vi "find_point_in_tables.vi"(8 "T No.":enum16{"0", "1", "2", "3", "4"}(ring), 9 "T Search":dbl, 10 "P Search":dbl) -> (3 "Point":T7)   [LabVIEW 2017]
uses:
  <vilib>/Utility/file.llb/Read Delimited Spreadsheet (DBL).vi
panel:
  out "all rows":dbl[][](array[numeric])
  out "appended path":path
  out "P Search 2":dbl
  out "T Founded":dbl
  out "Super_Heated_T_Curves":T1(ring)
  out "Super_Heated_S_Curves":enum16{"P", "S", "H gas"}(ring)
  out "Super_Heated_T_Curves 2":T2
  out "Super_Heated_S_Curves 2":T3
  out "Sat_Deg_10_Step":T4(ring)
  out "Sat_Deg_10_Step 2":T5
  out "Sat_By_Deg":T4(ring)
  out "Sat_By_Deg 2":T6
  out "Saturation Degrees( 10 Steps )":dbl[][](array[numeric])
  out "Super_Heated_S_Curves 3":dbl[][](array[numeric])
  out "Super_Heated_T":dbl[][](array[numeric])
  out "T Search Index In Sat Table":dbl
  out "Sat_By_Deg_Arr":dbl[][](array[numeric])
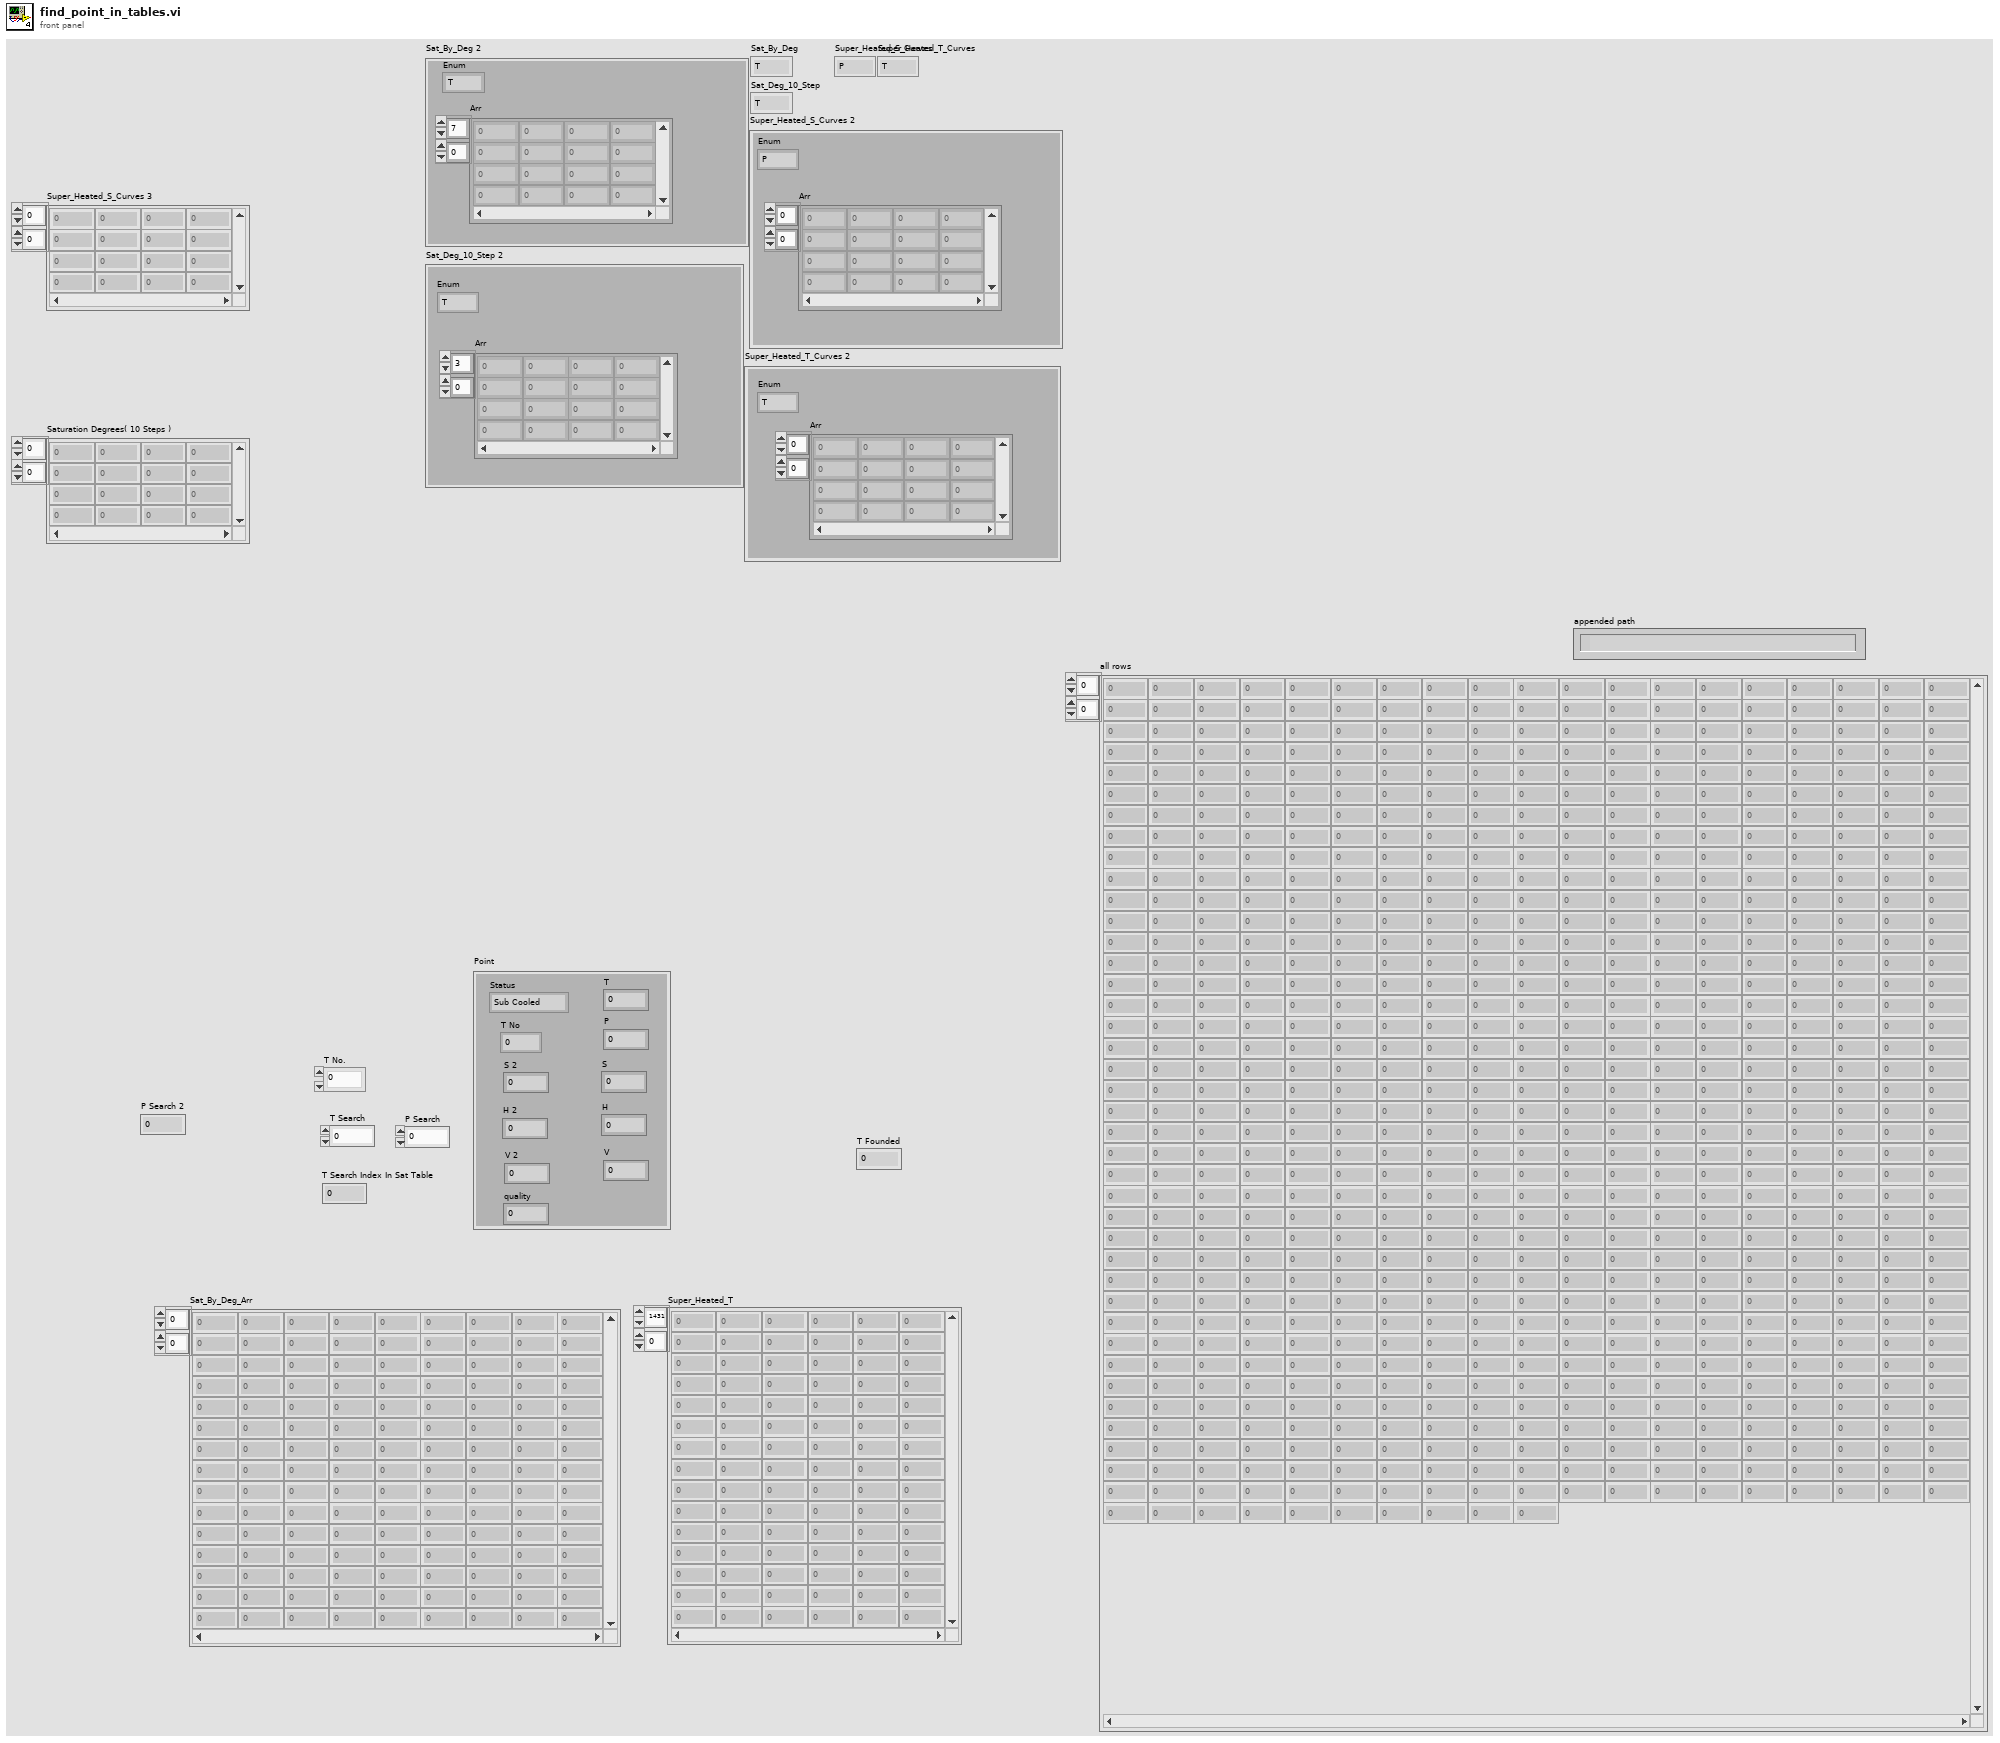
[diagram p1: front panel]
types:
  T1 = enum16{"T", "P", "T_Sat_Vapor", "Hg", "Sg", "Vg"}
  T2 = cluster{"Enum":enum16{"T", "P", "T_Sat_Vapor", "Hg", "Sg", "Vg"}, "Arr":dbl[][]}
  T3 = cluster{"Enum":enum16{"P", "S", "H gas"}, "Arr":dbl[][]}
  T4 = enum16{"T", "P", "V1", "Vg", "H1", "Hg", "R", "S1", "Sg"}
  T5 = cluster{"Enum":enum16{"T", "P", "V1", "Vg", "H1", "Hg", "R", "S1", "Sg"}, "Arr":dbl[][]}
  T6 = cluster{"Enum":enum16{"T", "P", "V1", "Vg", "H1", "Hg", "R", "S1", "Sg"}, "Arr ":dbl[][]}
  T7 = cluster{"S":dbl, "H":dbl, "V":dbl, "T":dbl, "P":dbl, "Status":enum16{"Sub Cooled", "Saturation", "Super Heated"}, "S 2":dbl, "H 2":dbl, "V 2":dbl, "T No":enum16{"0", "1", "2", "3", "4"}, "quality":dbl}
  T8 = enum16{"Sub Cooled", "Saturation", "Super Heated"}
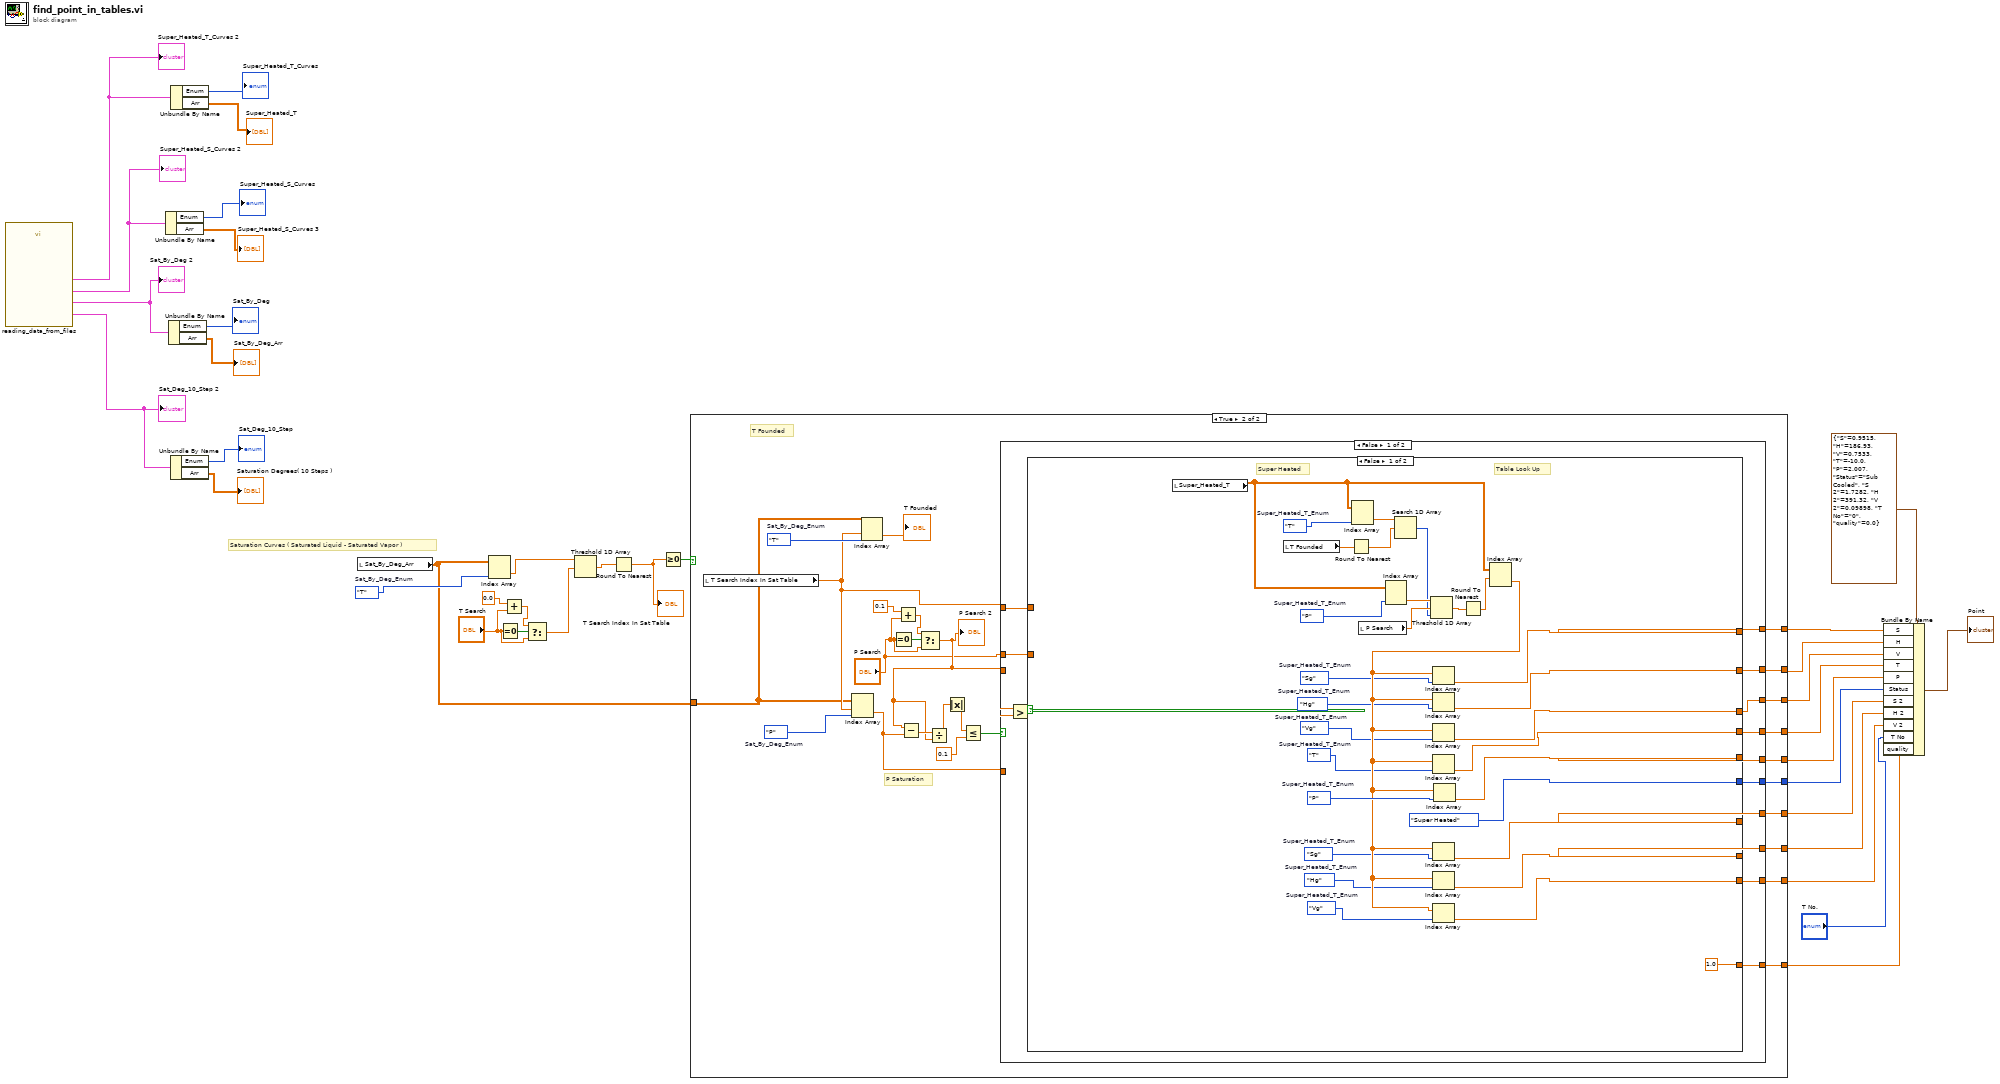
[diagram p0: block diagram]
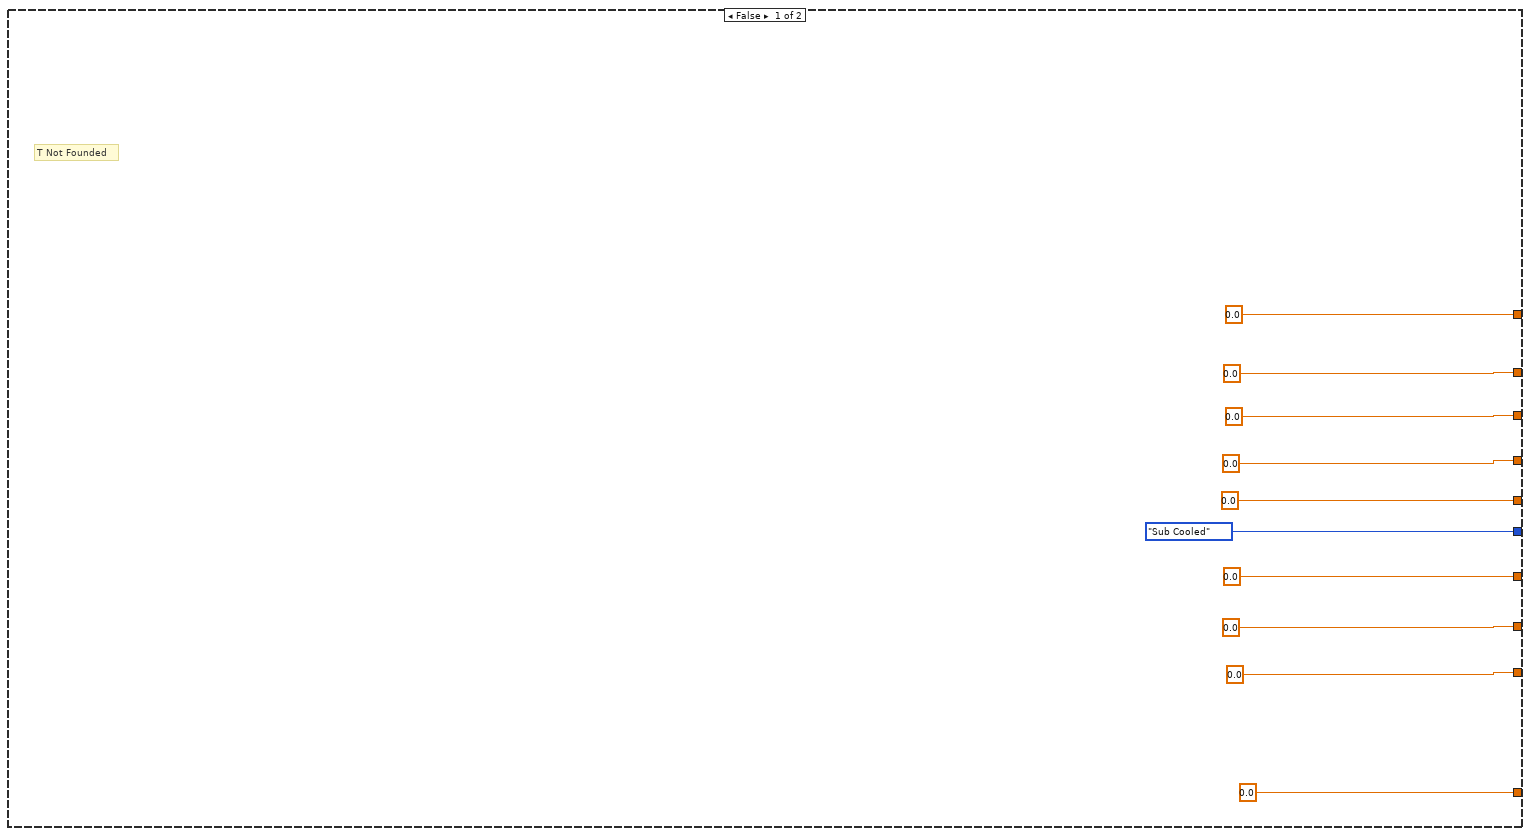
[diagram p2: hidden frame]
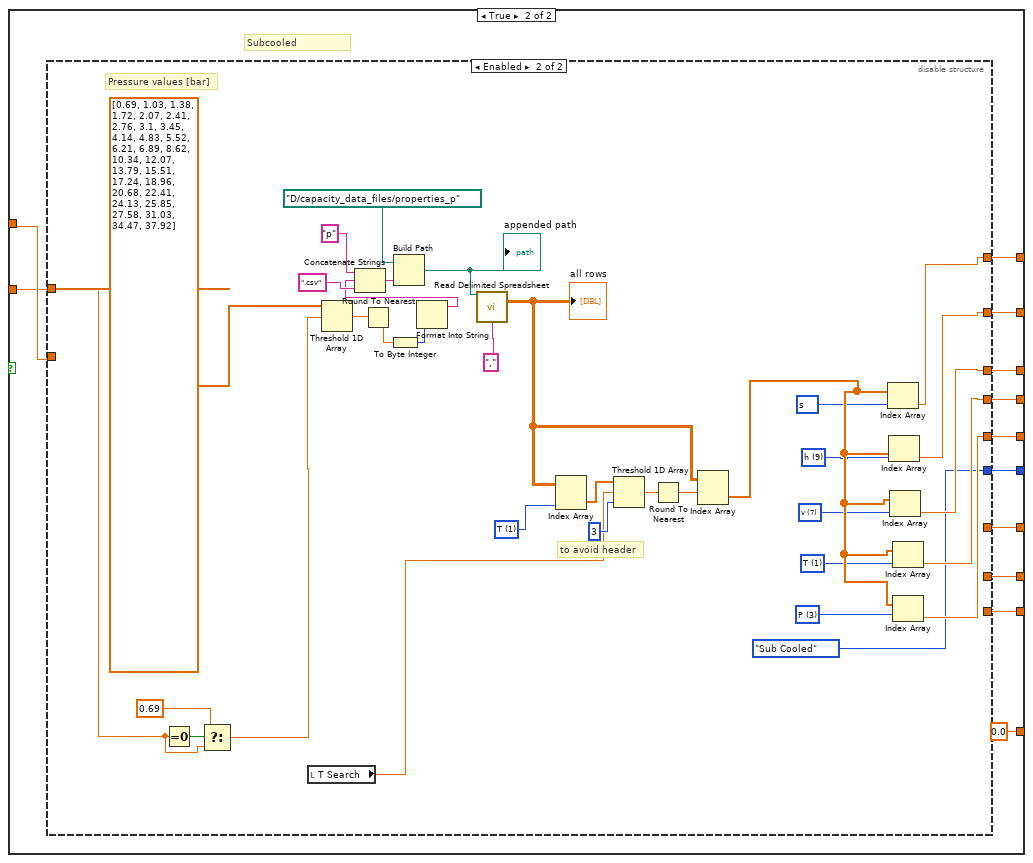
[diagram p3: hidden frame]
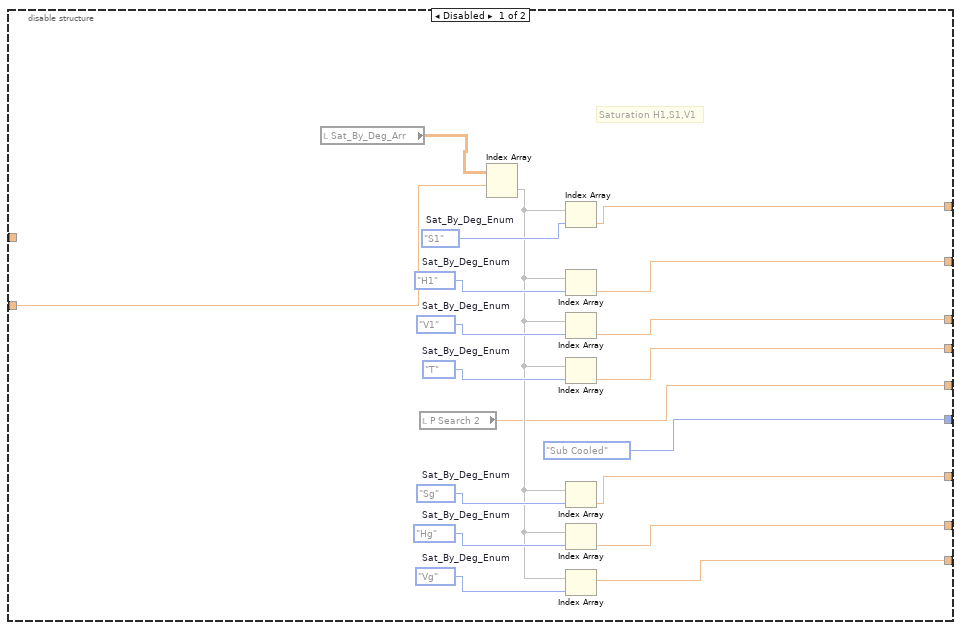
[diagram p4: hidden frame]
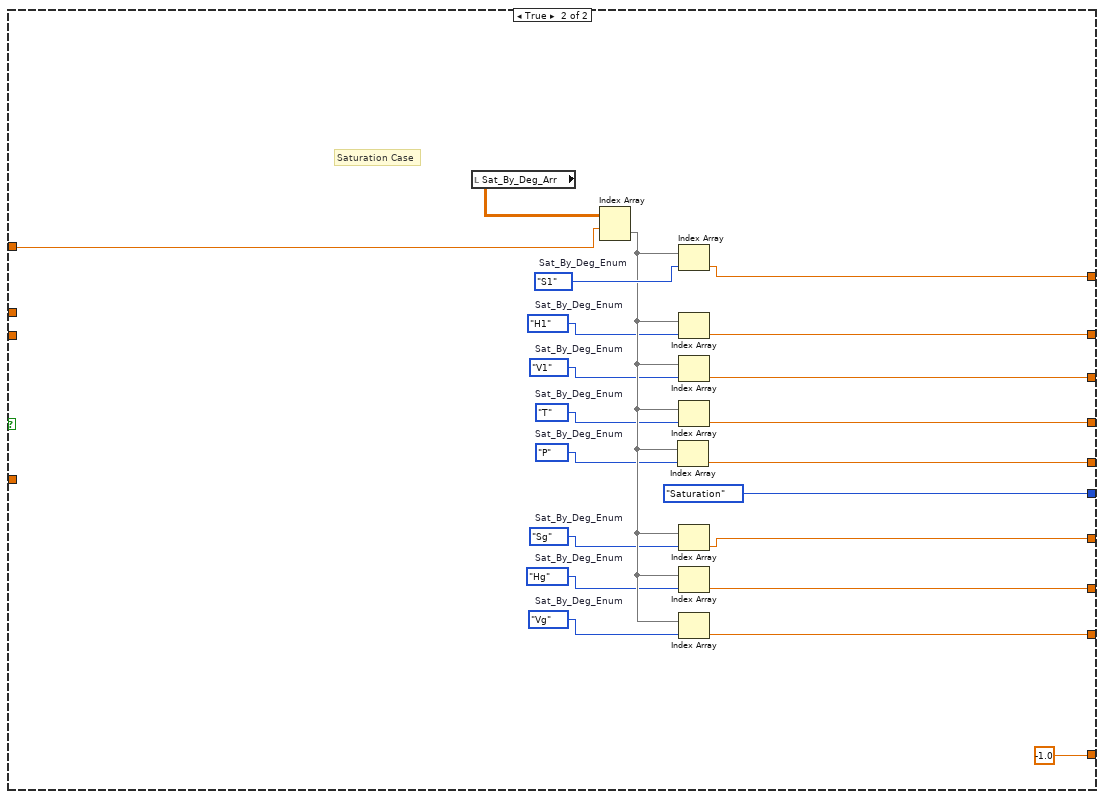
[diagram p5: hidden frame]
diagram:
  w34 = T4."T"  # Sat_By_Deg_Enum
  # "Saturation Curves ( Saturated Liquid - Saturated Vapor )"
  n1 = call "reading_data_from_files.vi"() -> ("Super_Heated_T_Curves"=w14:T2, "Super_Heated_S_Curves"=w15:T3, "Sat_Deg_10_Step"=w18:T5, "Sat_By_Deg"=w20:T6)  [unwired: 8 in]
  "Sat_By_Deg 2" <- w20
  "Sat_Deg_10_Step 2" <- w18
  "Super_Heated_S_Curves 2" <- w15
  "Super_Heated_T_Curves 2" <- w14
  n2 = Unbundle By Name(w15) -> ("Enum"=→"Super_Heated_S_Curves":enum16{"P", "S", "H gas"}, "Arr"=→"Super_Heated_S_Curves 3":dbl[][])
  n3 = Unbundle By Name(w20) -> ("Enum"=→"Sat_By_Deg":T4, "Arr"=→"Sat_By_Deg_Arr":dbl[][])
  n4 = Unbundle By Name(w18) -> ("Enum"=→"Sat_Deg_10_Step":T4, "Arr"=→"Saturation Degrees( 10 Steps )":dbl[][])
  n5 = Unbundle By Name(w14) -> ("Enum"=→"Super_Heated_T_Curves":T1, "Arr"=→"Super_Heated_T":dbl[][])
  n6 = local read "Sat_By_Deg_Arr"() -> (w22:dbl[][])
  n7 = Index Array(array=w22, index (col)=w34) -> (element=w24:dbl[])  [unwired: 1 in]
  n8 = Equal To 0?(x="T Search") -> (x = 0?=w7:bool)
  n9 = Add(x=0.0, y="T Search") -> (x+y=w6:dbl)
  n10 = Select(t=w6, s=w7, f="T Search") -> (s? t:f=w3:dbl)
  n11 = Threshold 1D Array(2:w3, 3:w24) -> (0:w23:dbl)  [unwired: 1 in]
  n12 = Round To Nearest(number=w23) -> (nearest integer value=w21:dbl)
  "T Search Index In Sat Table" <- w21
  n13 = Greater Or Equal To 0?(x=w21) -> (x >= 0?=w36:bool)
  n14 = case shown="True" w36 {
    tunnel: [0.0 ("Numeric") w72] -> w33
    tunnel: [0.0 ("Numeric") w71] -> w32
    tunnel: [0.0 ("Numeric") w70] -> w31
    tunnel: [0.0 ("Numeric") w69] -> w30
    tunnel: [0.0 ("Numeric") w68] -> w29
    tunnel: [0.0 ("Numeric") w67] -> w28
    tunnel: [0.0 ("Numeric") w66] -> w27
    tunnel: [0.0 ("Numeric") w65] -> w26
    tunnel: [T8."Sub Cooled" ("Status") w64] -> w25
    tunnel: w22 -> [_ w57]
    tunnel: [0.0 w47] -> w1
    frame False {
      # "T Not Founded"
    }
    frame True {
      w59 = T4."T"  # Sat_By_Deg_Enum
      w63 = T4."P"  # Sat_By_Deg_Enum
      # "P Saturation"
      # "T Founded"
      n15 = local read "T Search Index In Sat Table"() -> (w58:dbl)
      n16 = Index Array(array=w57, index (row)=w58, index (col)=w63) -> (element=w60:dbl)
      n17 = Index Array(array=w57, index (row)=w58, index (col)=w59) -> (element=→"T Founded":dbl)
      n18 = Equal To 0?(x="P Search") -> (x = 0?=w52:bool)
      n19 = Add(x=0.1, y="P Search") -> (x+y=w51:dbl)
      n20 = Select(t=w51, s=w52, f="P Search") -> (s? t:f=w49:dbl)
      "P Search 2" <- w49
      n21 = Subtract(x=w49, y=w60) -> (x-y=w55:dbl)
      n22 = Divide(x=w55, y=w49) -> (x/y=w54:dbl)
      n23 = Absolute Value(x=w54) -> (abs(x)=w53:dbl)
      n24 = Less Or Equal?(x=w53, y=0.1) -> (x <= y?=w61:bool)
      n25 = case shown="False" w61 {
        tunnel: w58 -> [w86 w202]
        tunnel: [w85 w192] -> w72
        tunnel: [w84 w191] -> w71
        tunnel: [w83 w190] -> w70
        tunnel: [w82 w189] -> w69
        tunnel: [w81 w188] -> w68
        tunnel: [w79 w187] -> w67
        tunnel: [w78 w186] -> w66
        tunnel: [w77 w185] -> w65
        tunnel: [w80 T8."Saturation" ("Status")] -> w64
        tunnel: w49 -> [w76 _]
        tunnel: w60 -> [w75 _]
        tunnel: "P Search" -> [w74 _]
        tunnel: [w73 -1.0] -> w47
        frame False {
          n26 = Greater?(x=w76, y=w75) -> (0:w87:bool)
          n27 = case shown="False" w87 {
            tunnel: w86 -> [_ w129]
            tunnel: [w103 w128] -> w85
            tunnel: [w102 w127] -> w84
            tunnel: [w101 w126] -> w83
            tunnel: [w100 w125] -> w82
            tunnel: [w99 w120] -> w81
            tunnel: [T8."Super Heated" ("Status") w124] -> w80
            tunnel: [w97 w123] -> w79
            tunnel: [w96 w122] -> w78
            tunnel: [w95 w121] -> w77
            tunnel: w74 -> [_ w119]
            tunnel: [1.0 0.0] -> w73
            frame False {
              w94 = T1."T"  # Super_Heated_T_Enum
              w112 = T1."P"  # Super_Heated_T_Enum
              w110 = T1."Vg"  # Super_Heated_T_Enum
              w109 = T1."Hg"  # Super_Heated_T_Enum
              w108 = T1."Sg"  # Super_Heated_T_Enum
              w107 = T1."T"  # Super_Heated_T_Enum
              w106 = T1."Vg"  # Super_Heated_T_Enum
              w105 = T1."Hg"  # Super_Heated_T_Enum
              w104 = T1."Sg"  # Super_Heated_T_Enum
              w117 = T1."P"  # Super_Heated_T_Enum
              # "Table Look Up"
              # "Super Heated"
              n28 = local read "Super_Heated_T"() -> (w91:dbl[][])
              n29 = local read "T Founded"() -> (w90:dbl)
              n30 = Round To Nearest(number=w90) -> (nearest integer value=w89:dbl)
              n31 = Index Array(array=w91, index (col)=w94) -> (element=w93:dbl[])  [unwired: 1 in]
              n32 = local read "P Search"() -> (w115:dbl)
              n33 = Index Array(array=w91, index (col)=w117) -> (element=w116:dbl[])  [unwired: 1 in]
              n34 = Search 1D Array(1D array=w93, element=w89) -> (index of element=w92:i32)  [unwired: 1 in]
              n35 = Threshold 1D Array(1:w92, 2:w115, 3:w116) -> (0:w114:dbl)
              n36 = Round To Nearest(number=w114) -> (nearest integer value=w113:dbl)
              n37 = Index Array(array=w91, index (row)=w113) -> (element=w111:dbl[])  [unwired: 1 in]
              n38 = Index Array(array=w111, index=w104) -> (element=w103:dbl)
              n39 = Index Array(array=w111, index=w105) -> (element=w102:dbl)
              n40 = Index Array(array=w111, index=w106) -> (element=w101:dbl)
              n41 = Index Array(array=w111, index=w107) -> (element=w100:dbl)
              n42 = Index Array(array=w111, index=w108) -> (element=w97:dbl)
              n43 = Index Array(array=w111, index=w109) -> (element=w96:dbl)
              n44 = Index Array(array=w111, index=w110) -> (element=w95:dbl)
              n45 = Index Array(array=w111, index=w112) -> (element=w99:dbl)
            }
            frame True {
              # "Subcooled"
              n46 = disable-structure shown="Enabled" {
                disable-tunnel: w129 -> [w140 _]
                disable-tunnel: [w139 w154] -> w128
                disable-tunnel: [w138 w153] -> w127
                disable-tunnel: [w137 w152] -> w126
                disable-tunnel: [w136 w151] -> w125
                disable-tunnel: [T8."Sub Cooled" ("Status") T8."Sub Cooled" ("Status")] -> w124
                disable-tunnel: [w134 _] -> w123
                disable-tunnel: [w133 _] -> w122
                disable-tunnel: [w132 _] -> w121
                disable-tunnel: [w130 w150] -> w120
                disable-tunnel: w119 -> [_ w181]
                frame Disabled {
                  w142 = T4."Vg"  # Sat_By_Deg_Enum
                  w143 = T4."Hg"  # Sat_By_Deg_Enum
                  w144 = T4."Sg"  # Sat_By_Deg_Enum
                  w145 = T4."T"  # Sat_By_Deg_Enum
                  w146 = T4."V1"  # Sat_By_Deg_Enum
                  w147 = T4."H1"  # Sat_By_Deg_Enum
                  w148 = T4."S1"  # Sat_By_Deg_Enum
                  # "Saturation H1,S1,V1"
                  n47 = local read "Sat_By_Deg_Arr"() -> (w141:dbl[][])
                  n48 = local read "P Search 2"() -> (w130:dbl)
                  n49 = Index Array(array=w141, index (row)=w140) -> (element=w131:dbl[])  [unwired: 1 in]
                  n50 = Index Array(array=w131, index=w148) -> (element=w139:dbl)
                  n51 = Index Array(array=w131, index=w147) -> (element=w138:dbl)
                  n52 = Index Array(array=w131, index=w146) -> (element=w137:dbl)
                  n53 = Index Array(array=w131, index=w145) -> (element=w136:dbl)
                  n54 = Index Array(array=w131, index=w144) -> (element=w134:dbl)
                  n55 = Index Array(array=w131, index=w143) -> (element=w133:dbl)
                  n56 = Index Array(array=w131, index=w142) -> (element=w132:dbl)
                }
                frame Enabled {
                  w177 = u16 1 items=["T"=1, "P"=3, "rho"=5, "v"=7, "h"=9, "s"=11] ("properties columns")
                  w168 = u16 1 items=["T"=1, "P"=3, "rho"=5, "v"=7, "h"=9, "s"=11] ("properties columns")
                  w175 = u16 3 items=["T"=1, "P"=3, "rho"=5, "v"=7, "h"=9, "s"=11] ("properties columns")
                  w176 = u16 9 items=["T"=1, "P"=3, "rho"=5, "v"=7, "h"=9, "s"=11] ("properties columns")
                  w174 = u16 7 items=["T"=1, "P"=3, "rho"=5, "v"=7, "h"=9, "s"=11] ("properties columns")
                  w173 = u16 11 items=["T"=1, "P"=3, "rho"=5, "v"=7, "h"=9, "s"=11] ("properties columns")
                  # "to avoid header"
                  # "Pressure values [bar]"
                  n57 = Equal To 0?(x=w181) -> (x = 0?=w182:bool)
                  n58 = Select(t=0.69, s=w182, f=w181) -> (s? t:f=w156:dbl)
                  n59 = local read "T Search"() -> (w155:dbl)
                  n60 = Threshold 1D Array(2:w156, 3:dbl[] [0.69, 1.03, 1.38, 1.72, 2.07, 2.41, 2.76, 3.1, 3.45, 4.14, 4.83, 5.52, 6.21, 6.89, 8.62, 10.34, 12.07, 13.79, 15.51, 17.24, 18.96, 20.68, 22.41, 24.13, 25.85, 27.58, 31.03, 34.47, 37.92]) -> (0:w158:dbl)  [unwired: 1 in]
                  n61 = Round To Nearest(number=w158) -> (nearest integer value=w165:dbl)
                  n62 = To Byte Integer(number=w165) -> (8bit integer=w166:i8)
                  n63 = Format Into String(w166) -> (resulting string=w162:string)  [unwired: 3 in, 1 out]
                  n64 = Concatenate Strings("p" ("string"), w162, ".csv" ("string")) -> (w160:string)
                  n65 = Build Path(base path=path "D:/capacity_data_files/properties_p", name or relative path=w160) -> (appended path=w164:path)
                  "appended path" <- w164
                  n66 = call-poly <vilib>:"Read Delimited Spreadsheet.vi"("file path (dialog if empty)"=w164, "delimiter (\\t)"="," ("delimiter (\\t)")) -> ("all rows"=w171:dbl[][])  [unwired: 8 in, 5 out]
                  "all rows" <- w171
                  n67 = Index Array(array=w171, index (col)=w168) -> (element=w169:dbl[])  [unwired: 1 in]
                  n68 = Threshold 1D Array(1:3 ("start index (0)"), 2:w155, 3:w169) -> (0:w170:dbl)
                  n69 = Round To Nearest(number=w170) -> (nearest integer value=w172:dbl)
                  n70 = Index Array(array=w171, index (row)=w172) -> (element=w178:dbl[])  [unwired: 1 in]
                  n71 = Index Array(array=w178, index=w173) -> (element=w154:dbl)
                  n72 = Index Array(array=w178, index=w176) -> (element=w153:dbl)
                  n73 = Index Array(array=w178, index=w174) -> (element=w152:dbl)
                  n74 = Index Array(array=w178, index=w177) -> (element=w151:dbl)
                  n75 = Index Array(array=w178, index=w175) -> (element=w150:dbl)
                }
              }
            }
          }
        }
        frame True {
          w193 = T4."Vg"  # Sat_By_Deg_Enum
          w194 = T4."Hg"  # Sat_By_Deg_Enum
          w195 = T4."Sg"  # Sat_By_Deg_Enum
          w196 = T4."P"  # Sat_By_Deg_Enum
          w197 = T4."T"  # Sat_By_Deg_Enum
          w198 = T4."V1"  # Sat_By_Deg_Enum
          w199 = T4."H1"  # Sat_By_Deg_Enum
          w201 = T4."S1"  # Sat_By_Deg_Enum
          # "Saturation Case"
          n76 = local read "Sat_By_Deg_Arr"() -> (w203:dbl[][])
          n77 = Index Array(array=w203, index (row)=w202) -> (element=w200:dbl[])  [unwired: 1 in]
          n78 = Index Array(array=w200, index=w196) -> (element=w188:dbl)
          n79 = Index Array(array=w200, index=w201) -> (element=w192:dbl)
          n80 = Index Array(array=w200, index=w199) -> (element=w191:dbl)
          n81 = Index Array(array=w200, index=w198) -> (element=w190:dbl)
          n82 = Index Array(array=w200, index=w197) -> (element=w189:dbl)
          n83 = Index Array(array=w200, index=w195) -> (element=w187:dbl)
          n84 = Index Array(array=w200, index=w194) -> (element=w186:dbl)
          n85 = Index Array(array=w200, index=w193) -> (element=w185:dbl)
        }
      }
    }
  }
  n86 = Bundle By Name(cluster=T7 {"S"=0.9515, "H"=186.93, "V"=0.7533, "T"=-10.0, "P"=2.007, "Status"=enum."Sub Cooled", "S 2"=1.7282, "H 2"=391.32, "V 2"=0.09898, "T No"=enum."0", "quality"=0.0} ("Point 2"), "S"=w33, "H"=w32, "V"=w31, "T"=w30, "P"=w29, "Status"=w25, "S 2"=w28, "H 2"=w27, "V 2"=w26, "T No"="T No.", "quality"=w1) -> (→"Point":T7)
